vi "test CompactSubObj.vi"(11 "Test Case In":refnum<class "test Electronic Datasheet.lvclass">) -> (0 "error out":errorcluster, 3 "Test Case Out":refnum<class "test Electronic Datasheet.lvclass">)   [LabVIEW 2024, in "test Electronic Datasheet.lvclass"]
uses:
  test Electronic Datasheet.lvclass
  test Electronic Datasheet.lvclass/test Electronic Datasheet.ctl
  4993e8ee-a06a-463a-9684-69129f64d5ce.vi
  Electronic Datasheet/Electronic Datasheet.lvclass
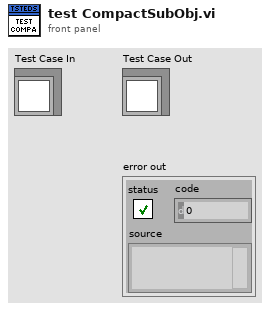
[diagram p1: front panel]
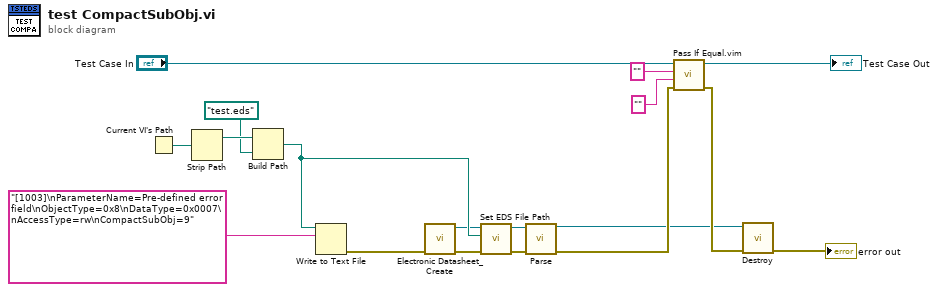
[diagram p0: block diagram]
diagram:
  n1 = Current VI's Path() -> (path=w12:path)
  n2 = Strip Path(path=w12) -> (stripped path=w11:path)  [unwired: 1 out]
  n3 = Build Path(base path=w11, name or relative path=path "test.eds") -> (appended path=w7:path)
  n4 = Write to Text File(file (use dialog)=w7, text="[1003]\nParameterName=Pre-defined error field\nObjectType=0x8\nDataType=0x0007\nAccessType=rw\nCompactSubObj=9") -> (error out=w9:errorcluster)  [unwired: 2 in, 2 out]
  n5 = call "Electronic Datasheet_Create.vi"("Error In"=w9) -> ("Error Out"=w5:errorcluster, "reference out"=w4:refnum<class "Electronic Datasheet.lvclass">)  [unwired: 9 in]
  n6 = call "Set EDS File Path.vi"("EDS File Path"=w7, "reference in"=w4) -> ("reference out"=w8:refnum<class "Electronic Datasheet.lvclass">)  [unwired: 8 in, 1 out]
  n7 = call "Parse.vi"("error in"=w5, "reference in"=w8) -> ("error out"=w14:errorcluster, "reference out"=w1:refnum<class "Electronic Datasheet.lvclass">)  [unwired: 8 in]
  n8 = call "Pass If Equal.vim"("error in (no error)"=w14, "Actual"="", "Expected"="", "LUnit Test Case In"="Test Case In") -> ("error out"=w3:errorcluster, "LUnit Test Case Out"=→"Test Case Out":refnum<class "test Electronic Datasheet.lvclass">)  [unwired: 6 in]
  n9 = call-dynamic "Destroy.vi"("Error In"=w3, "reference in"=w1) -> ("Error Out"=→"error out":errorcluster)  [unwired: 8 in, 1 out]
